vi "Case structures 2.vi"() -> ()   [LabVIEW 2022 SP3]
panel:
  out "error out":errorcluster
  out "Weather Data Out":T1
  in  "error in":errorcluster
  in  "Weather Data In":T1
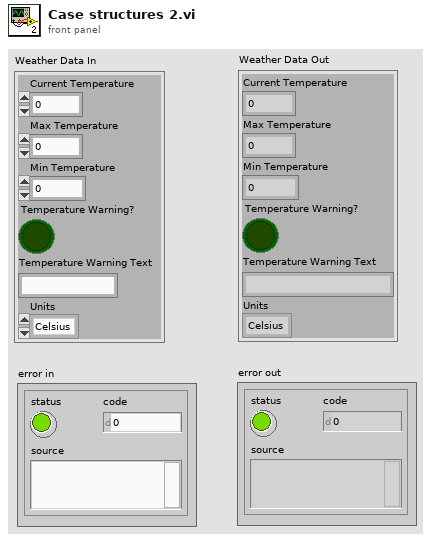
[diagram p1: front panel]
types:
  T1 = cluster{"Current Temperature":dbl, "Max Temperature":dbl, "Min Temperature":dbl, "Temperature Warning?":bool, "Temperature Warning Text":string, "Units":enum16{"Celsius", "Fahrenheit"}}
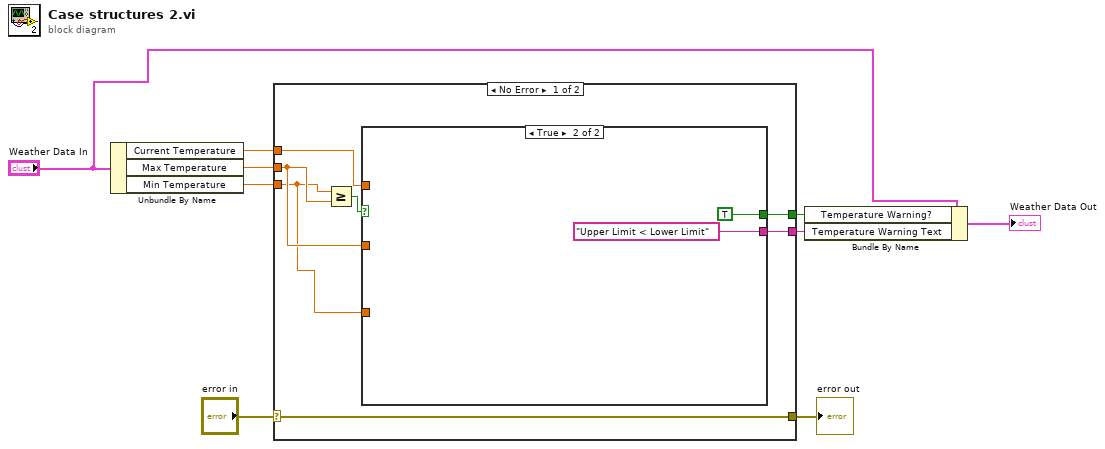
[diagram p0: block diagram]
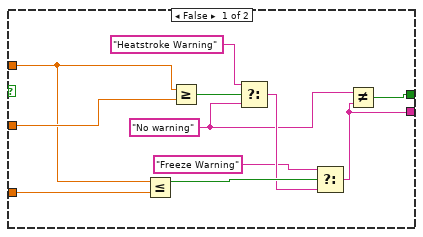
[diagram p2: hidden frame]
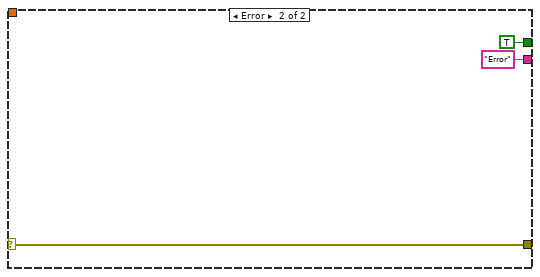
[diagram p3: hidden frame]
diagram:
  n1 = Unbundle By Name "Unbundle By Name"("Weather Data In") -> ("Current Temperature"=w6:dbl, "Max Temperature"=w7:dbl, "Min Temperature"=w8:dbl)
  n2 = case shown="No Error" "error in" {
    selector: "error in" -> [w11 w32]
    tunnel: w8 -> [w10 _]
    tunnel: w7 -> [w14 _]
    tunnel: w6 -> [w15 _]
    tunnel: [w13 TRUE ("Temperature Warning?")] -> w3
    tunnel: [w12 "Error" ("Temperature Warning Text")] -> w2
    tunnel: [w11 w32] -> w1
    frame No Error {
      n3 = Greater Or Equal?(x=w10, y=w14) -> (x >= y?=w16:bool)
      n4 = case shown="True" w16 {
        tunnel: w15 -> [w24 _]
        tunnel: w14 -> [w27 _]
        tunnel: [w19 TRUE ("Temperature Warning?")] -> w13
        tunnel: [w18 "Upper Limit < Lower Limit" ("Temperature Warning Text")] -> w12
        tunnel: w10 -> [w17 _]
        frame False {
          w20 = "No warning"
          n5 = Less Or Equal?(x=w24, y=w17) -> (x <= y?=w23:bool)
          n6 = Greater Or Equal?(x=w24, y=w27) -> (x >= y?=w26:bool)
          n7 = Select(t="Heatstroke Warning", s=w26, f=w20) -> (s? t:f=w22:string)
          n8 = Select(t="Freeze Warning", s=w23, f=w22) -> (s? t:f=w18:string)
          n9 = Not Equal?(x=w20, y=w18) -> (x != y?=w19:bool)
        }
        frame True {
        }
      }
    }
    frame Error {
    }
  }
  "error out" <- w1
  n10 = Bundle By Name(cluster="Weather Data In", "Temperature Warning?"=w3, "Temperature Warning Text"=w2) -> (→"Weather Data Out":T1)
